vi "niRFUtil RFHS Math Complex Magnitude.vi"(0 "data in":csg[](array[numeric]), 2 "RFHS?":bool=TRUE, 7 "result in":sgl[](array[numeric]), 11 "error in":errorcluster) -> (4 "result out":sgl[](array[numeric]), 15 "error out":errorcluster)   [LabVIEW 2015, in "niRFUtil.lvlib"]
uses:
  niRFUtil.lvlib
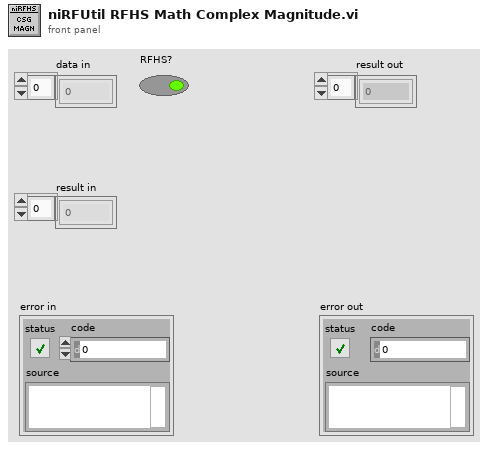
[diagram p1: front panel]
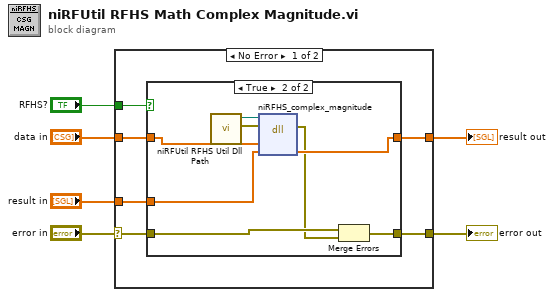
[diagram p0: block diagram]
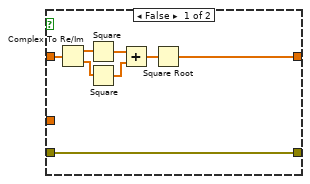
[diagram p2: hidden frame]
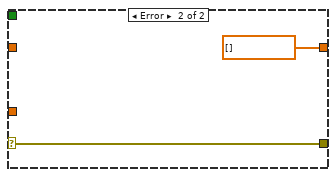
[diagram p3: hidden frame]
diagram:
  n1 = case shown="No Error" "error in" {
    selector: "error in" -> [w9 w30]
    tunnel: "RFHS?" -> [w12 _]
    tunnel: "data in" -> [w11 _]
    tunnel: [w10 sgl[] [] ("result")] -> w4
    tunnel: [w8 w30] -> w2
    tunnel: "result in" -> [w7 _]
    frame No Error {
      n2 = case shown="True" w12 {
        tunnel: w11 -> [w14 w28]
        tunnel: [w13 w27] -> w10
        tunnel: w9 -> [w20 w24]
        tunnel: [w20 w22] -> w8
        tunnel: w7 -> [_ w21]
        frame False {
          n3 = Complex To Re/Im(x + iy=w14) -> (x=w16:sgl[], y=w15:sgl[])
          n4 = Square(x=w16) -> (x^2=w19:sgl[])
          n5 = Square(x=w15) -> (x^2=w18:sgl[])
          n6 = Add(x=w19, y=w18) -> (x+y=w17:sgl[])
          n7 = Square Root(x=w17) -> (sqrt(x)=w13:sgl[])
        }
        frame True {
          n8 = call "niRFUtil RFHS Util Dll Path.vi"() -> ("error out"=w26:errorcluster, "Path"=w25:path)  [unwired: 7 in, 3 out]
          n9 = dll-call lib="R:/niRFHS.dll" fn="niRFHS_complex_magnitude"(path in=w25, error in=w26, "data"=w28, "result"=w21) -> (error out=w23:errorcluster, "result"=w27:sgl[])  [unwired: 3 in, 1 out]
          n10 = Merge Errors(w24, w23) -> (w22:errorcluster)
        }
      }
    }
    frame Error {
    }
  }
  "result out" <- w4
  "error out" <- w2
